vi "Set VI Properties to Force FP to Load.vi"(8 "error in (no error)":errorcluster, 11 "VI in":refnum<vi>) -> (0 "error out":errorcluster, 3 "VI out":refnum<vi>)   [LabVIEW 2020]
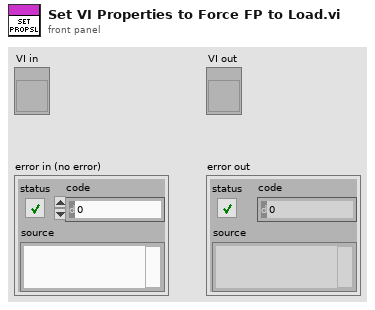
[diagram p1: front panel]
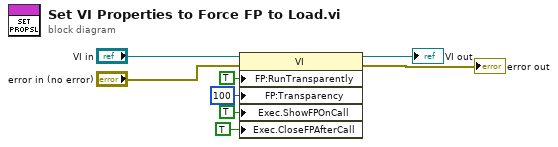
[diagram p0: block diagram]
diagram:
  n1 = property class="VI"(reference="VI in", error in="error in (no error)", "FP:RunTransparently"=TRUE ("Front Panel Window:Run VI Transparently"), "FP:Transparency"=u8 100 ("Front Panel Window:Transparency"), "Exec.ShowFPOnCall"=TRUE ("Execution:Show Front Panel On Call"), "Exec.CloseFPAfterCall"=TRUE ("Execution:Close After Call")) -> (reference out=→"VI out":refnum<vi>, error out=→"error out":errorcluster)
